vi "UART_Str_Timeout.vi"(6 "行数量":u32, 8 "error in (no error)":errorcluster caption="错误输入（无错误）", 9 "超时s":dbl=0.1, 10 "写入字符串":string=">01 *idn?\n>01 *idn?", 11 "BASE_COM":refnum<visa-resource-name>="COM1") -> (0 "error out":errorcluster caption="错误输出", 1 "OK":bool, 2 "读取字符串":string, 3 "BASE_COM_OUT":refnum<visa-resource-name>, 4 "等待时间ms":u32)   [LabVIEW 2015, in "UARTCOM.lvlib"]
uses:
  UARTCOM.lvlib
  <vilib>/Utility/error.llb/Error Cluster From Error Code.vi
  <vilib>/ErrorRing/Error Ring.xnode
panel:
  # "行数量设为0时，则依据写入字符串行数量来确定返回数据行数"
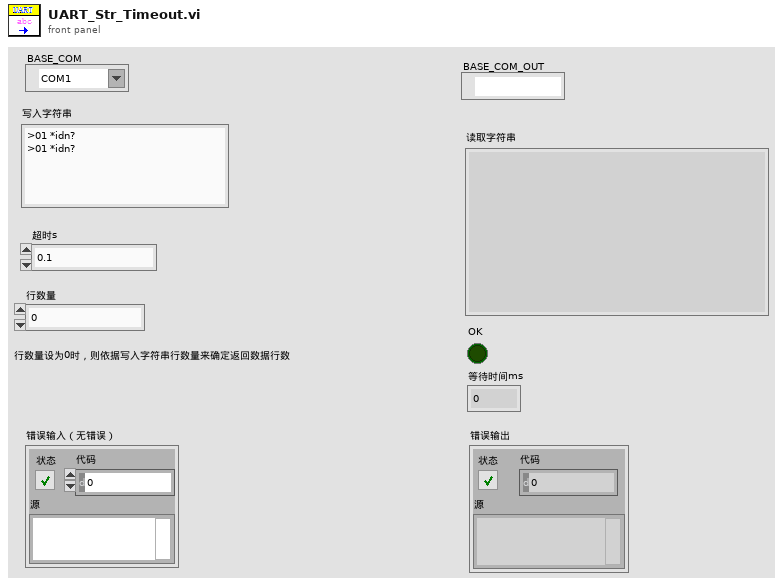
[diagram p1: front panel]
types:
  T1 = typedef "Semaphore RefNum" = refnum<k1>
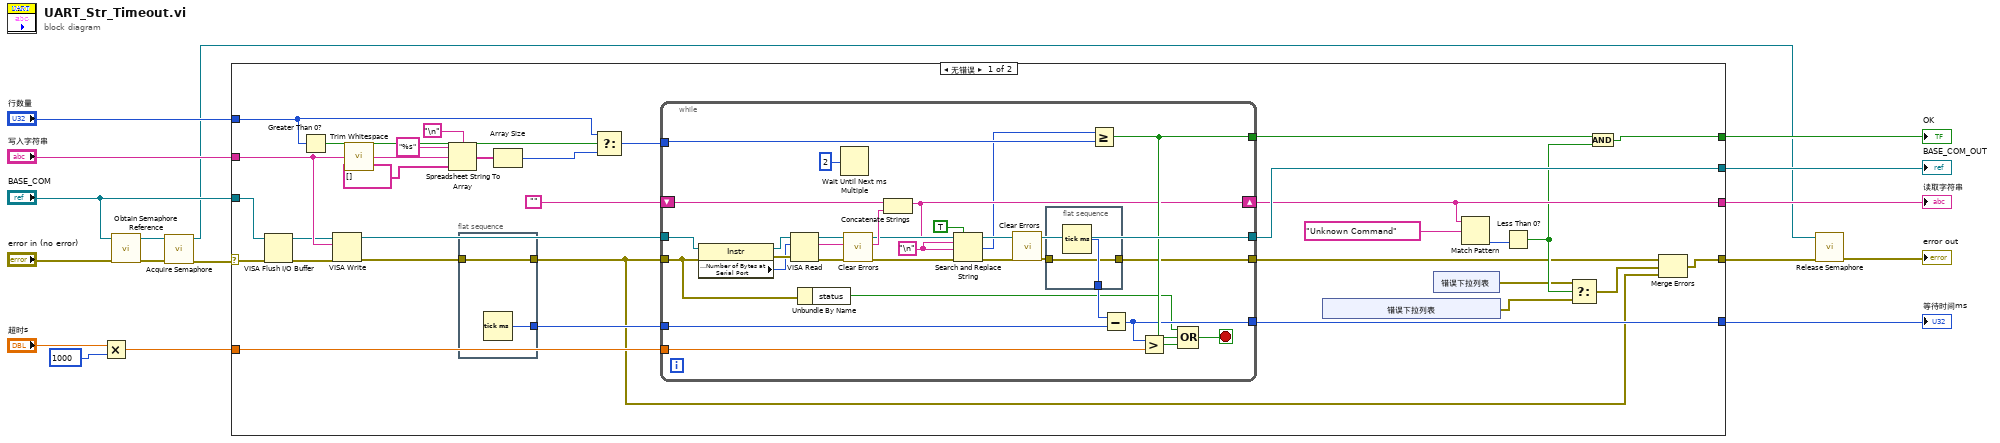
[diagram p0: block diagram]
diagram:
  n1 = Multiply(x="超时s", y=1000) -> (x*y=w13:dbl)
  n2 = call <vilib>:"Obtain Semaphore Reference.vi"("error in (no error)"="error in (no error)", "name (unnamed)"="BASE_COM") -> ("error out"=w6:errorcluster, "semaphore"=w5:T1)  [unwired: 3 in, 1 out]
  n3 = call <vilib>:"Acquire Semaphore.vi"("error in (no error)"=w6, "semaphore"=w5) -> ("error out"=w3:errorcluster, "semaphore out"=w4:T1)  [unwired: 3 in, 1 out]
  n4 = case shown="无错误" w3 {
    selector: w3 -> [w37 w88]
    tunnel: "BASE_COM" -> [w35 w89]
    tunnel: [w40 w89] -> w17
    tunnel: [w25 w88] -> w2
    tunnel: "写入字符串" -> [w50 _]
    tunnel: w13 -> [w43 _]
    tunnel: [w31 _] -> w12
    tunnel: [w29 _] -> w11
    tunnel: [w39 _] -> w10
    tunnel: "行数量" -> [w22 _]
    frame No Error {
      n5 = VISA Flush I/O Buffer(VISA resource name=w35, error in (no error)=w37) -> (VISA resource name out=w34:refnum<visa-resource-name>, error out=w36:errorcluster)  [unwired: 1 in]
      n6 = Greater Than 0?(x=w22) -> (x > 0?=w23:bool)
      n7 = VISA Write(VISA resource name=w34, write buffer=w50, error in (no error)=w36) -> (VISA resource name out=w42:refnum<visa-resource-name>, error out=w38:errorcluster)  [unwired: 1 out]
      n8 = call <vilib>:"Trim Whitespace.vi"("string"=w50) -> ("trimmed string"=w48:string)  [unwired: 1 in]
      n9 = Spreadsheet String To Array(delimiter (Tab)="\n", format string="%s", spreadsheet string=w48, array type (2D Dbl)=string[] []) -> (array=w45:string[])
      n10 = flat-sequence {
        tunnel: [w58] -> w44
        tunnel: w38 -> [w57]
        tunnel: [w57] -> w20
        frame #0 {
          n11 = Tick Count (ms)() -> (millisecond timer value=w58:u32)
        }
      }
      n12 = Array Size(array=w45) -> (size(s)=w24:i32)
      n13 = Select(t=w22, s=w23, f=w24) -> (s? t:f=w21:u32)
      n14 = while {
        tunnel: w21 -> [w78]
        tunnel: w44 -> [w85]
        tunnel: w43 -> [w84]
        tunnel: w20 -> [w63]
        tunnel: w42 -> [w68]
        shift-right: [w76] -> w31
        shift-left: "" -> [w81]
        tunnel: [w79] -> w40
        tunnel: [w77] -> w30
        tunnel: [w71] -> w27
        tunnel: [w72] -> w39
        stop <- w82 stop-if-true
        w75 = "\n"
        n15 = property class="Instr"(reference=w68, error in=w63) -> (reference out=w67:refnum<visa-resource-name>, error out=w69:errorcluster, "Serial Settings:Number of Bytes at Serial Port"=w66:u32)
        n16 = VISA Read(VISA resource name=w67, byte count=w66, error in (no error)=w69) -> (VISA resource name out=w79:refnum<visa-resource-name>, read buffer=w80:string, error out=w61:errorcluster)  [unwired: 1 out]
        n17 = Unbundle By Name(w63) -> ("status"=w62:bool)
        n18 = Wait Until Next ms Multiple(millisecond multiple=u32 2 ("毫秒倍数")) -> ()  [unwired: 1 out]
        n19 = call <vilib>:"Clear Errors.vi"("error in (no error)"=w61) -> ("error out"=w60:errorcluster)  [unwired: 5 in, 1 out]
        n20 = Concatenate Strings(w81, w80) -> (w76:string)
        n21 = Search and Replace String(replace all?=TRUE ("替换全部？(F)"), input string=w76, search string=w75, replace string=w75, error in=w60) -> (number of replacements=w73:i32, error out=w65:errorcluster)  [unwired: 3 in, 2 out]
        n22 = call <vilib>:"Clear Errors.vi"("error in (no error)"=w65) -> ("error out"=w64:errorcluster)  [unwired: 5 in, 1 out]
        n23 = flat-sequence {
          tunnel: [w87] -> w70
          tunnel: w64 -> [w86]
          tunnel: [w86] -> w71
          frame #0 {
            n24 = Tick Count (ms)() -> (millisecond timer value=w87:u32)
          }
        }
        n25 = Greater Or Equal?(x=w73, y=w78) -> (x >= y?=w77:bool)
        n26 = Subtract(x=w70, y=w85) -> (x-y=w72:u32)
        n27 = Greater?(x=w72, y=w84) -> (0:w83:bool)
        n28 = Compound Arithmetic op=OR ("复合运算")(w62, w77, w83) -> (w82:bool)
      }
      n29 = xnode "错误下拉列表"() -> ("错误输出"=w18:errorcluster)
      n30 = xnode "错误下拉列表"() -> ("错误输出"=w19:errorcluster)
      n31 = Match Pattern(string=w31, regular expression="Unknown Command") -> (offset past match=w33:i32)  [unwired: 1 in, 3 out]
      n32 = Less Than 0?(x=w33) -> (x < 0?=w28:bool)
      n33 = Select(t=w19, s=w28, f=w18) -> (s? t:f=w26:errorcluster)
      n34 = And(x=w30, y=w28) -> (x .and. y?=w29:bool)
      n35 = Merge Errors(w27, w26, w20) -> (w25:errorcluster)
    }
    frame Error {
    }
  }
  "BASE_COM_OUT" <- w17
  "读取字符串" <- w12
  "OK" <- w11
  "等待时间ms" <- w10
  n36 = call <vilib>:"Release Semaphore.vi"("error in (no error)"=w2, "semaphore"=w4) -> ("error out"=→"error out":errorcluster)  [unwired: 4 in, 1 out]
